vi "信号发生器3.0【波形图表】.vi"() -> ()   [LabVIEW 2022 SP3]
uses:
  <vilib>/Analysis/baseanly.llb/Mean (DBL).vi
  <vilib>/measure/NI_MABase.lvlib
  <vilib>/measure/NI_MAPro.lvlib
  <vilib>/Analysis/NI_AALBase.lvlib
panel:
  out "开始指示灯":bool
  out "波形图表":waveform(dbl)(graph)
  out "波形信息":string
  in  "信号发生器开关":bool
  out "采集结束指示灯":bool
  out "波形编号":i64
  out "程序中止指示灯":bool
  out "中间类型":string
  out "中间保存数组":dbl[](array[numeric])
  in  "保存":bool
  out "算数平均值":dbl
  out "最小值":dbl
  out "最大值":dbl
  in  "停止":bool
  in  "保存路径":path
  in  "自定义公式":string
  in  "采样数":i64(slide) scale=1.0..1000.0
  in  "采样率":i64(slide) scale=150.0..1500.0
  in  "偏移量":i64(knob) scale=-5.0..5.0
  in  "标准差\n（高斯白噪声）":dbl(knob) scale=0.0..1.0
  in  "幅度":i64(knob) scale=0.0..10.0
  in  "频率":dbl(knob) scale=0.0..1.0
  in  "波形类型":u16(ring) items=["三角波", "正弦波", "自定义波形", "方波", "锯齿波"]
  # "信号发生器   MZ-0016"
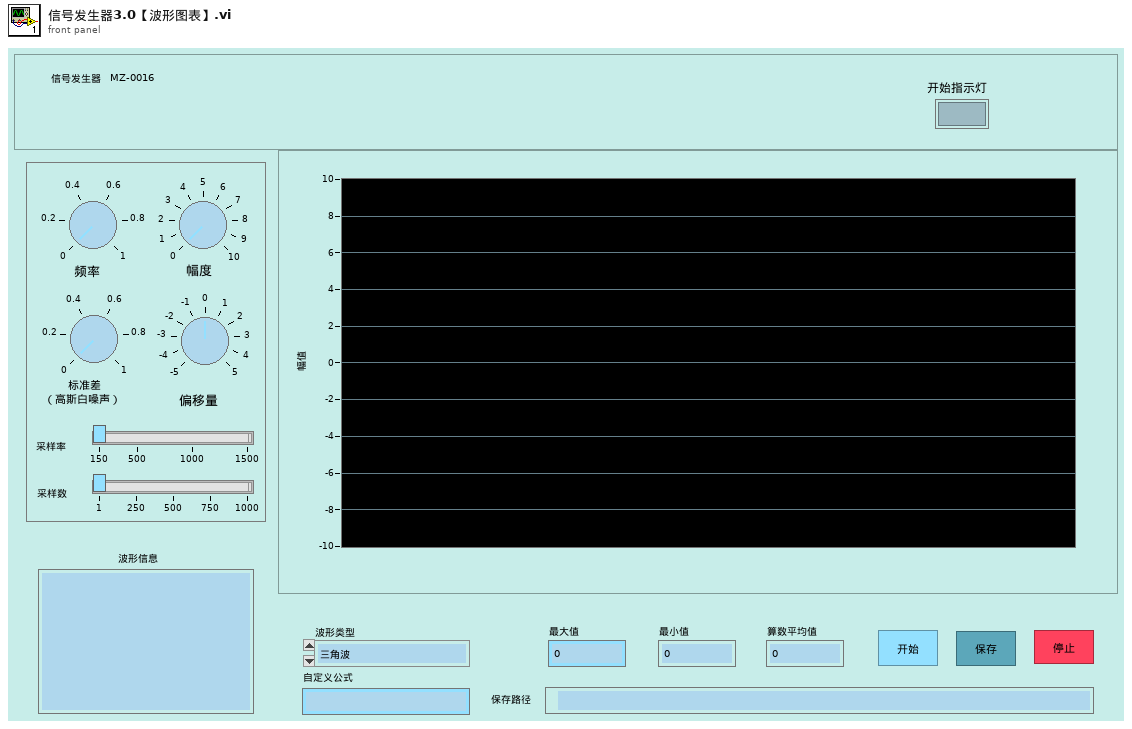
[diagram p1: front panel]
types:
  T1 = enum16{"open", "replace", "create", "open or create", "replace or create", "replace or create with confirmation"}
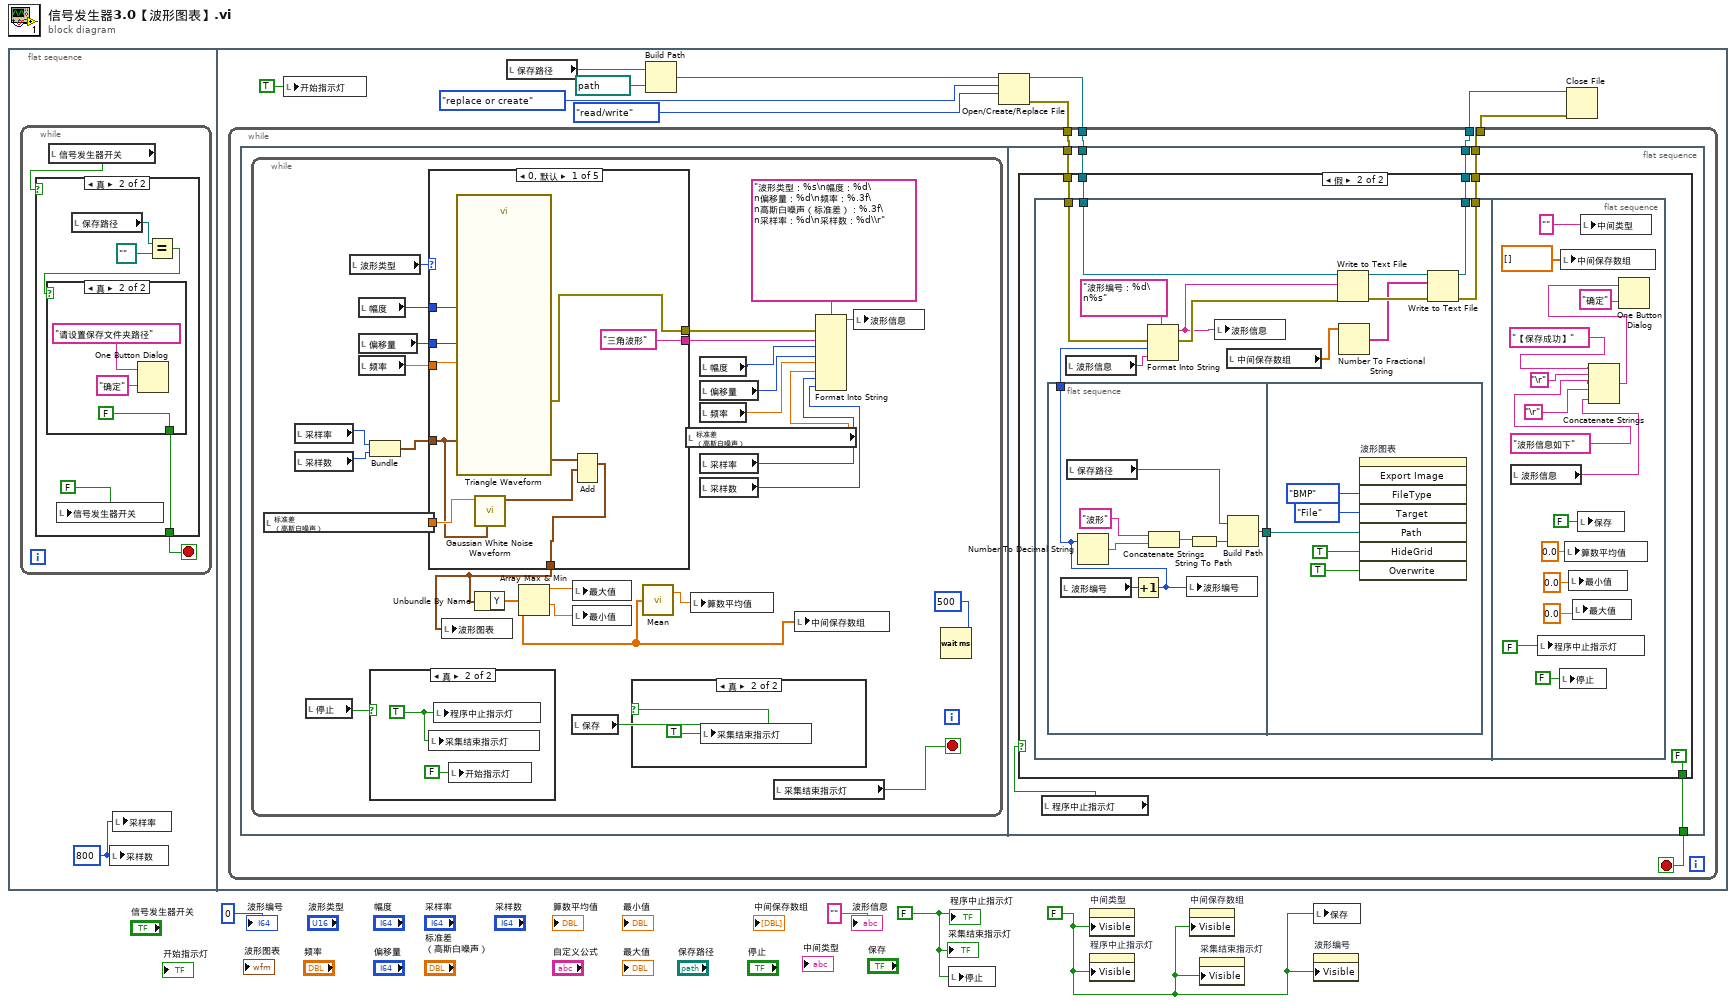
[diagram p0: block diagram]
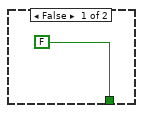
[diagram p2: hidden frame]
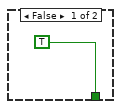
[diagram p3: hidden frame]
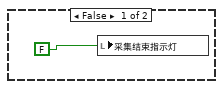
[diagram p4: hidden frame]
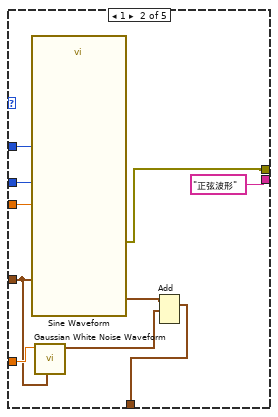
[diagram p6: hidden frame]
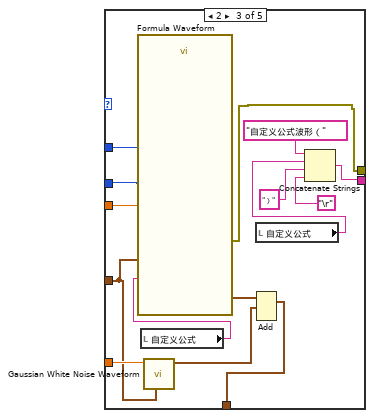
[diagram p7: hidden frame]
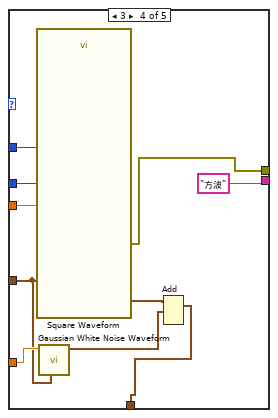
[diagram p8: hidden frame]
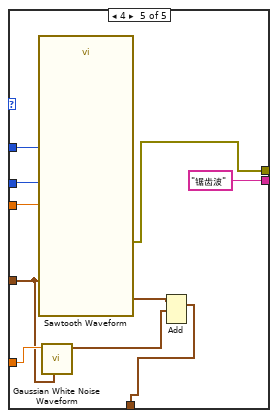
[diagram p9: hidden frame]
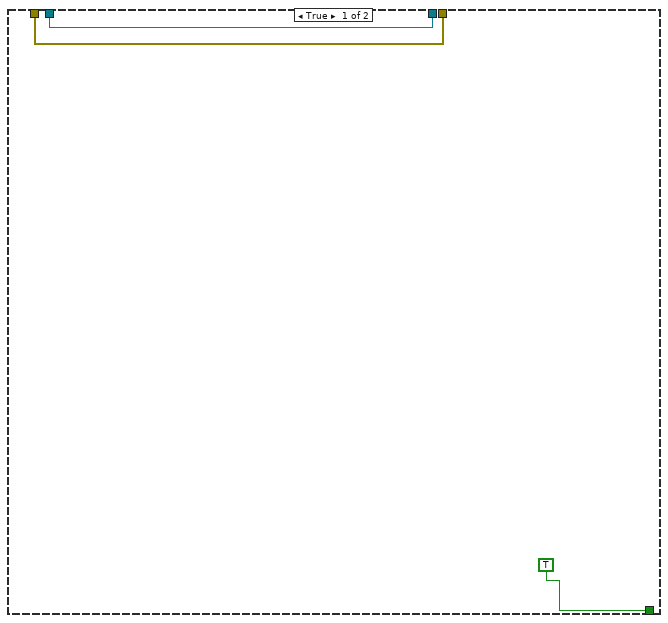
[diagram p10: hidden frame]
diagram:
  w2 = FALSE
  w1 = FALSE ("可见")
  n1 = flat-sequence {
    frame #0 {
      w5 = i64 800 ("采样数")
      n2 = while {
        stop <- w6 stop-if-true
        n3 = local read "信号发生器开关"() -> (w7:bool)
        n4 = case shown="真" w7 {
          tunnel: [FALSE w10] -> w6
          frame False {
          }
          frame True {
            n5 = local write "信号发生器开关"(FALSE) -> ()
            n6 = local read "保存路径"() -> (w13:path)
            n7 = Equal?(x=w13, y=path "") -> (x = y?=w11:bool)
            n8 = case shown="真" w11 {
              tunnel: [TRUE FALSE] -> w10
              frame False {
              }
              frame True {
                n9 = One Button Dialog(message="请设置保存文件夹路径" ("消息"), button name ("OK")="确定" ("按钮名称（“确定”）")) -> ()  [unwired: 1 out]
              }
            }
          }
        }
      }
      n10 = local write "采样数"(w5) -> ()
      n11 = local write "采样率"(w5) -> ()
    }
    frame #1 {
      n12 = local write "开始指示灯"(TRUE ("开始指示灯")) -> ()
      n13 = local read "保存路径"() -> (w19:path)
      n14 = Build Path(base path=w19, name or relative path=path "记录.txt") -> (appended path=w26:path)
      n15 = Open/Create/Replace File(file path (use dialog)=w26, operation (0:open)=T1."replace or create" ("操作(0:open)"), access (0:read/write)=enum16{"read/write", "read-only", "write-only"}."read/write" ("权限(0:read/write)")) -> (refnum out=w22:refnum<file>, error out=w23:errorcluster)  [unwired: 3 in, 1 out]
      n16 = while {
        tunnel: w23 -> [w29]
        tunnel: w22 -> [w28]
        tunnel: [w32] -> w21
        tunnel: [w31] -> w20
        stop <- w30 stop-if-true
        n17 = flat-sequence {
          tunnel: w28 -> [w124]
          tunnel: [w123] -> w32
          tunnel: [w122] -> w31
          tunnel: [w119] -> w30
          tunnel: w29 -> [w120]
          frame #0 {
            n18 = while {
              stop <- w33 stop-if-true
              n19 = local read "标准差\n（高斯白噪声）"() -> (w58:dbl)
              n20 = local read "采样率"() -> (w54:i64)
              n21 = local read "采样数"() -> (w53:i64)
              n22 = local read "停止"() -> (w34:bool)
              n23 = local read "波形类型"() -> (w59:u16)
              n24 = local read "幅度"() -> (w55:i64)
              n25 = local read "偏移量"() -> (w56:i64)
              n26 = local read "频率"() -> (w57:dbl)
              n27 = Bundle("采样率"=w54, "采样数"=w53) -> (w52:cluster{"采样率":i64, "采样数":i64})  [unwired: 1 in]
              n28 = case shown="真" w34 {
                frame False {
                }
                frame True {
                  w63 = TRUE ("程序中止指示灯")
                  n29 = local write "采集结束指示灯"(w63) -> ()
                  n30 = local write "程序中止指示灯"(w63) -> ()
                  n31 = local write "开始指示灯"(FALSE ("开始指示灯")) -> ()
                }
              }
              n32 = case shown="0, 默认" w59 {
                tunnel: w58 -> [w70 w80 w93 w102 w113]
                tunnel: w57 -> [w71 w81 w98 w105 w114]
                tunnel: w56 -> [w72 w82 w97 w104 w115]
                tunnel: w55 -> [w73 w83 w96 w103 w116]
                tunnel: w52 -> [w69 w79 w92 w101 w111]
                tunnel: [w66 w76 w86 w106 w112] -> w36
                tunnel: ["三角波形" "正弦波形" w85 "方波" "锯齿波"] -> w39
                tunnel: [w64 w74 w84 w99 w109] -> w38
                frame 0, Default {
                  n33 = call <vilib>:"Triangle Waveform.vi"("offset"=w72, "sampling info"=w69, "amplitude"=w73, "frequency"=w71) -> ("error out"=w64:errorcluster, "signal out"=w68:waveform(dbl))  [unwired: 6 in]
                  n34 = call <vilib>:"Gaussian White Noise Waveform.vi"("sampling info"=w69, "standard deviation"=w70) -> ("signal out"=w67:waveform(dbl))  [unwired: 8 in, 1 out]
                  n35 = Add(1:w67, 2:w68) -> (0:w66:waveform(dbl))  [unwired: 1 in, 1 out]
                }
                frame 1 {
                  n36 = call <vilib>:"Sine Waveform.vi"("offset"=w82, "sampling info"=w79, "amplitude"=w83, "frequency"=w81) -> ("error out"=w74:errorcluster, "signal out"=w78:waveform(dbl))  [unwired: 6 in]
                  n37 = call <vilib>:"Gaussian White Noise Waveform.vi"("sampling info"=w79, "standard deviation"=w80) -> ("signal out"=w77:waveform(dbl))  [unwired: 8 in, 1 out]
                  n38 = Add(1:w77, 2:w78) -> (0:w76:waveform(dbl))  [unwired: 1 in, 1 out]
                }
                frame 2 {
                  n39 = local read "自定义公式"() -> (w95:string)
                  n40 = call <vilib>:"Formula Waveform.vi"("offset"=w97, "sampling info"=w92, "formula"=w95, "amplitude"=w96, "frequency"=w98) -> ("error out"=w84:errorcluster, "signal out"=w94:waveform(dbl))  [unwired: 5 in]
                  n41 = call <vilib>:"Gaussian White Noise Waveform.vi"("sampling info"=w92, "standard deviation"=w93) -> ("signal out"=w91:waveform(dbl))  [unwired: 8 in, 1 out]
                  n42 = Add(1:w91, 2:w94) -> (0:w86:waveform(dbl))  [unwired: 1 in, 1 out]
                  n43 = local read "自定义公式"() -> (w89:string)
                  n44 = Concatenate Strings("自定义公式波形（", w89, "）" ("字符串"), "\r") -> (w85:string)
                }
                frame 3 {
                  n45 = call <vilib>:"Square Waveform.vi"("offset"=w104, "sampling info"=w101, "amplitude"=w103, "frequency"=w105) -> ("error out"=w99:errorcluster, "signal out"=w108:waveform(dbl))  [unwired: 6 in]
                  n46 = call <vilib>:"Gaussian White Noise Waveform.vi"("sampling info"=w101, "standard deviation"=w102) -> ("signal out"=w107:waveform(dbl))  [unwired: 8 in, 1 out]
                  n47 = Add(1:w107, 2:w108) -> (0:w106:waveform(dbl))  [unwired: 1 in, 1 out]
                }
                frame 4 {
                  n48 = call <vilib>:"Sawtooth Waveform.vi"("offset"=w115, "sampling info"=w111, "amplitude"=w116, "frequency"=w114) -> ("error out"=w109:errorcluster, "signal out"=w118:waveform(dbl))  [unwired: 6 in]
                  n49 = call <vilib>:"Gaussian White Noise Waveform.vi"("sampling info"=w111, "standard deviation"=w113) -> ("signal out"=w117:waveform(dbl))  [unwired: 8 in, 1 out]
                  n50 = Add(1:w117, 2:w118) -> (0:w112:waveform(dbl))  [unwired: 1 in, 1 out]
                }
              }
              n51 = local write "波形图表"(w36) -> ()
              n52 = Unbundle By Name(w36) -> ("Y"=w48:dbl[])
              n53 = Array Max & Min(array=w48) -> (max value=w49:dbl, min value=w50:dbl)  [unwired: 2 out]
              n54 = local read "保存"() -> (w35:bool)
              n55 = local write "最大值"(w49) -> ()
              n56 = local write "最小值"(w50) -> ()
              n57 = case shown="真" w35 {
                frame False {
                  n58 = local write "采集结束指示灯"(FALSE) -> ()
                }
                frame True {
                  n59 = local write "采集结束指示灯"(TRUE) -> ()
                }
              }
              n60 = call-poly <vilib>:"Mean.vi"("X"=w48) -> ("mean"=w51:dbl)  [unwired: 1 out]
              n61 = local read "标准差\n（高斯白噪声）"() -> (w45:dbl)
              n62 = local write "算数平均值"(w51) -> ()
              n63 = local read "幅度"() -> (w42:i64)
              n64 = local read "偏移量"() -> (w43:i64)
              n65 = local read "频率"() -> (w44:dbl)
              n66 = local read "采样率"() -> (w46:i64)
              n67 = local read "采样数"() -> (w47:i64)
              n68 = local read "采集结束指示灯"() -> (w33:bool)
              n69 = local write "中间保存数组"(w48) -> ()
              n70 = Format Into String(format string="波形类型：%s\n幅度：%d\n偏移量：%d\n频率：%.3f\n高斯白噪声（标准差）：%.3f\n采样率：%d\n采样数：%d\\r", error in=w38, w39, w42, w43, w44, w45, w46, w47) -> (resulting string=w40:string)  [unwired: 1 in, 1 out]
              n71 = local write "波形信息"(w40) -> ()
              n72 = Wait (ms)(milliseconds to wait=u32 500 ("毫秒计时值")) -> ()  [unwired: 1 out]
            }
          }
          frame #1 {
            n73 = local read "程序中止指示灯"() -> (w121:bool)
            n74 = case shown="假" w121 {
              tunnel: w124 -> [w127 w132]
              tunnel: w120 -> [w126 w131]
              tunnel: [w126 w130] -> w123
              tunnel: [w127 w129] -> w122
              tunnel: [TRUE FALSE] -> w119
              frame True {
              }
              frame False {
                n75 = flat-sequence {
                  tunnel: w132 -> [w146]
                  tunnel: w131 -> [w137]
                  tunnel: [w142] -> w130
                  tunnel: [w141] -> w129
                  frame #0 {
                    n76 = flat-sequence {
                      tunnel: [w152] -> w139
                      tunnel: [w147] -> w136
                      tunnel: w139 -> [w159]
                      frame #0 {
                        n77 = local read "波形编号"() -> (w154:i64)
                        n78 = local read "保存路径"() -> (w153:path)
                        n79 = Increment(x=w154) -> (x+1=w147:i64)
                        n80 = Number To Decimal String(number=w147) -> (decimal integer string=w150:string)  [unwired: 1 in]
                        n81 = Concatenate Strings("波形" ("连接的字符串"), w150) -> (w149:string)
                        n82 = local write "波形编号"(w147) -> ()
                        n83 = String To Path(string=w149) -> (path=w151:path)
                        n84 = Build Path(base path=w153, name or relative path=w151) -> (appended path=w152:path)
                      }
                      frame #1 {
                        n85 = invoke on="波形图表" class="WFChart (严格)" method="Export Image"("FileType"=enum32{"BMP", "EPS", "EMF", "PICT"}."BMP" ("文件类型"), "Target"=enum32{"File", "Clipboard"}."File" ("目标"), "Path"=w159, "HideGrid"=TRUE ("隐藏网格"), "Overwrite"=TRUE ("始终覆盖")) -> ()  [unwired: 3 in, 8 out]
                      }
                    }
                    n86 = local read "波形信息"() -> (w135:string)
                    n87 = Format Into String(format string="波形编号：%d\n%s", error in=w137, w136, w135) -> (resulting string=w133:string, error out=w134:errorcluster)  [unwired: 1 in]
                    n88 = local write "波形信息"(w133) -> ()
                    n89 = local read "中间保存数组"() -> (w140:dbl[])
                    n90 = Write to Text File(file (use dialog)=w146, text=w133, error in=w134) -> (refnum out=w145:refnum<file>, error out=w144:errorcluster)  [unwired: 1 in, 1 out]
                    n91 = Number To Fractional String(number=w140) -> (F-format string=w143:string[])  [unwired: 3 in]
                    n92 = Write to Text File(file (use dialog)=w145, text=w143, error in=w144) -> (refnum out=w141:refnum<file>, error out=w142:errorcluster)  [unwired: 1 in, 1 out]
                  }
                  frame #1 {
                    n93 = local read "波形信息"() -> (w161:string)
                    n94 = local write "程序中止指示灯"(FALSE) -> ()
                    n95 = local write "停止"(FALSE ("停止")) -> ()
                    n96 = local write "中间保存数组"(dbl[] [] ("中间保存数组")) -> ()
                    n97 = local write "算数平均值"(0.0 ("算数平均")) -> ()
                    n98 = local write "最小值"(0.0 ("最小值")) -> ()
                    n99 = local write "最大值"(0.0 ("最大值")) -> ()
                    n100 = local write "保存"(FALSE ("保存")) -> ()
                    n101 = local write "中间类型"("" ("中间类型字符串")) -> ()
                    n102 = Concatenate Strings("【保存成功】" ("消息"), "\r", "波形信息如下", "\r", w161) -> (w166:string)
                    n103 = One Button Dialog(message=w166, button name ("OK")="确定" ("按钮名称（“确定”）")) -> ()  [unwired: 1 out]
                  }
                }
              }
            }
          }
        }
      }
      n104 = Close File(refnum=w20, error in=w21) -> ()  [unwired: 2 out]
    }
  }
  n105 = local write "停止"(w2) -> ()
  n106 = property on="中间类型" class="Str"("Visible"=w1) -> ()  [unwired: 2 in, 2 out]
  n107 = property on="程序中止指示灯" class="Bool (严格)"("Visible"=w1) -> ()  [unwired: 2 in, 2 out]
  n108 = property on="中间保存数组" class="Arr (严格)"("Visible"=w1) -> ()  [unwired: 2 in, 2 out]
  n109 = property on="采集结束指示灯" class="Bool (严格)"("Visible"=w1) -> ()  [unwired: 2 in, 2 out]
  n110 = local write "保存"(w1) -> ()
  n111 = property on="波形编号" class="DigNum (严格)"("Visible"=w1) -> ()  [unwired: 2 in, 2 out]
  "程序中止指示灯" <- w2
  "波形编号" <- i64 0 ("波形编号")
  "波形信息" <- "" ("波形信息")
  "采集结束指示灯" <- w2
